vi "OpenPort.vi"(8 "error in (no error)":errorcluster caption="Fehler (Eingang, kein Fehler)", 11 "MoveoSerial Eingang":refnum<class "MoveoSerial.lvclass">) -> (0 "error out":errorcluster caption="Fehler (Ausgang)", 3 "MoveoSerial Ausgang":refnum<class "MoveoSerial.lvclass">)   [LabVIEW 2019, in "MoveoSerial.lvclass"]
uses:
  MoveoSerial.lvclass
  MoveoSerial.lvclass/MoveoSerial.ctl
  <vilib>/Instr/_visa.llb/VISA Configure Serial Port (Instr).vi
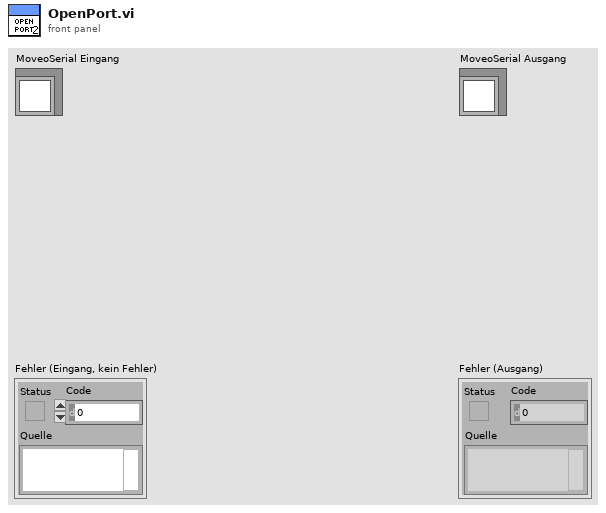
[diagram p1: front panel]
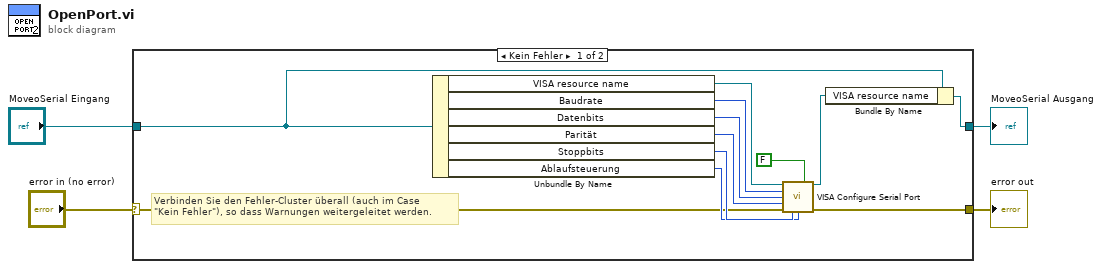
[diagram p0: block diagram]
diagram:
  n1 = case shown="Kein Fehler" "error in (no error)" {
    selector: "error in (no error)" -> [w7 w18]
    tunnel: [w6 w18] -> w3
    tunnel: [w9 w17] -> w1
    tunnel: "MoveoSerial Eingang" -> [w10 w17]
    frame No Error {
      # "Verbinden Sie den Fehler-Cluster überall (auch im Case\n\"Kein Fehler\"), so dass Warnungen weitergeleitet werden."
      n2 = Unbundle By Name(w10) -> ("VISA resource name"=w16:refnum<visa-resource-name>, "Baudrate"=w15:u32, "Datenbits"=w14:u16, "Parität"=w13:enum16{"None", "Odd", "Even", "Mark", "Space"}, "Stoppbits"=w12:u16, "Ablaufsteuerung"=w11:u16)
      n3 = call-poly "VISA Configure Serial Port"("VISA resource name"=w16, "Enable Termination\nChar (T)"=FALSE ("Enable Termination\nChar (T)"), "baud rate (9600)"=w15, "data bits (8)"=w14, "parity (0:none)"=w13, "error in (no error)"=w7, "stop bits (10: 1 bit)"=w12, "flow control (0:none)"=w11) -> ("VISA resource name out"=w8:refnum<visa-resource-name>, "error out"=w6:errorcluster)  [unwired: 2 in, 4 out]
      n4 = Bundle By Name(cluster=w10, "VISA resource name"=w8) -> (w9:refnum<class "MoveoSerial.lvclass">)
    }
    frame Error {
    }
  }
  "error out" <- w3
  "MoveoSerial Ausgang" <- w1
